vi "Get Controller .NET.vi"(11 "ControllerBase in":refnum<class "ControllerBase.lvclass">) -> (2 "ControllerBase":refnum<k24>, 3 "ControllerBase out":refnum<class "ControllerBase.lvclass">)   [LabVIEW 2025, in "ControllerBase.lvclass"]
uses:
  ControllerBase.lvclass
  D:/git/Sourcegrid-LabVIEW/dll/SourceGrid.dll
  dll/SourceGrid.dll
  ControllerBase.lvclass/ControllerBase.ctl
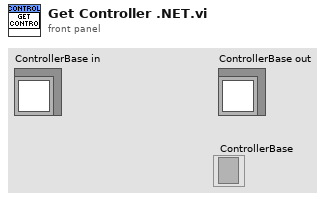
[diagram p1: front panel]
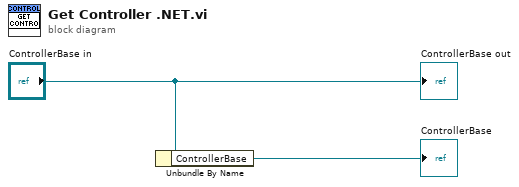
[diagram p0: block diagram]
diagram:
  n1 = Unbundle By Name("ControllerBase in") -> ("ControllerBase"=→"ControllerBase":refnum<k24>)
  "ControllerBase out" <- "ControllerBase in"
